vi "Read Spectrum and Save It.vi"(0 "VISA Session":refnum<visa-resource-name>, 6 "Pasta Destino DESTA aquisicao":path=path "d:/Users/Stinky/Documents", 9 "Corrente Atual (mA)":dbl, 11 "Error In":errorcluster, 12 "Iteracao":i32) -> (4 "Copy VISA Session":refnum<visa-resource-name>, 8 "PxI":dbl[](array[numeric]), 10 "XY Graph":T1(graph), 15 "Error Out":errorcluster)   [LabVIEW 2021]
uses:
  03b20bd4-ab24-4da3-90be-db98d83a5914.vi
panel:
  out "Return Data Bytes 2":u16
  out "Wavelike Data (X)":dbl[](array[numeric]) format="%.12f"
  out "Return All Data 2":string
  out "Wavelike Data (Y)":dbl[](array[numeric]) format="%.12f"
  out "Return Data Bytes":u16
  out "Return All Data":string
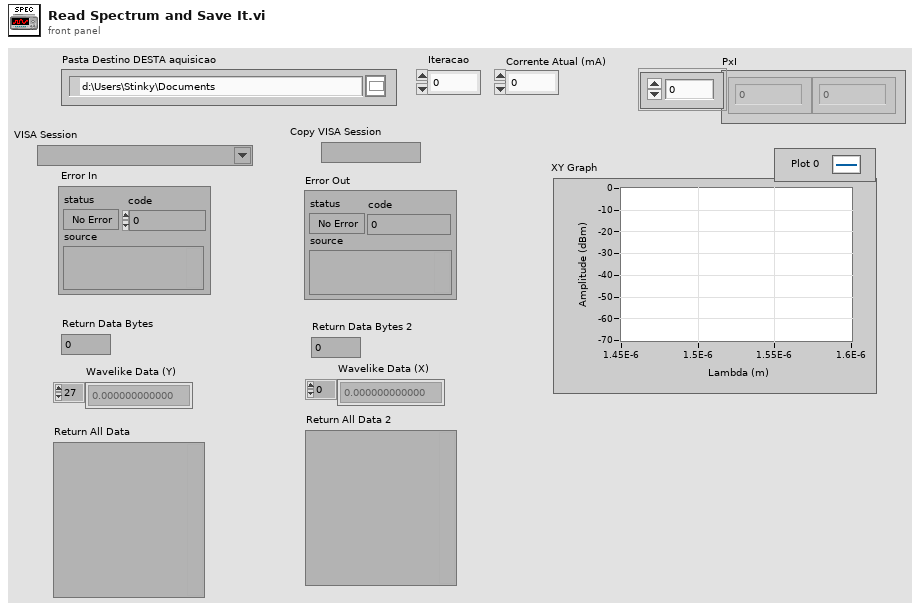
[diagram p1: front panel]
types:
  T1 = cluster{"Wavelike Data":dbl[], "Wavelike Data":dbl[]}
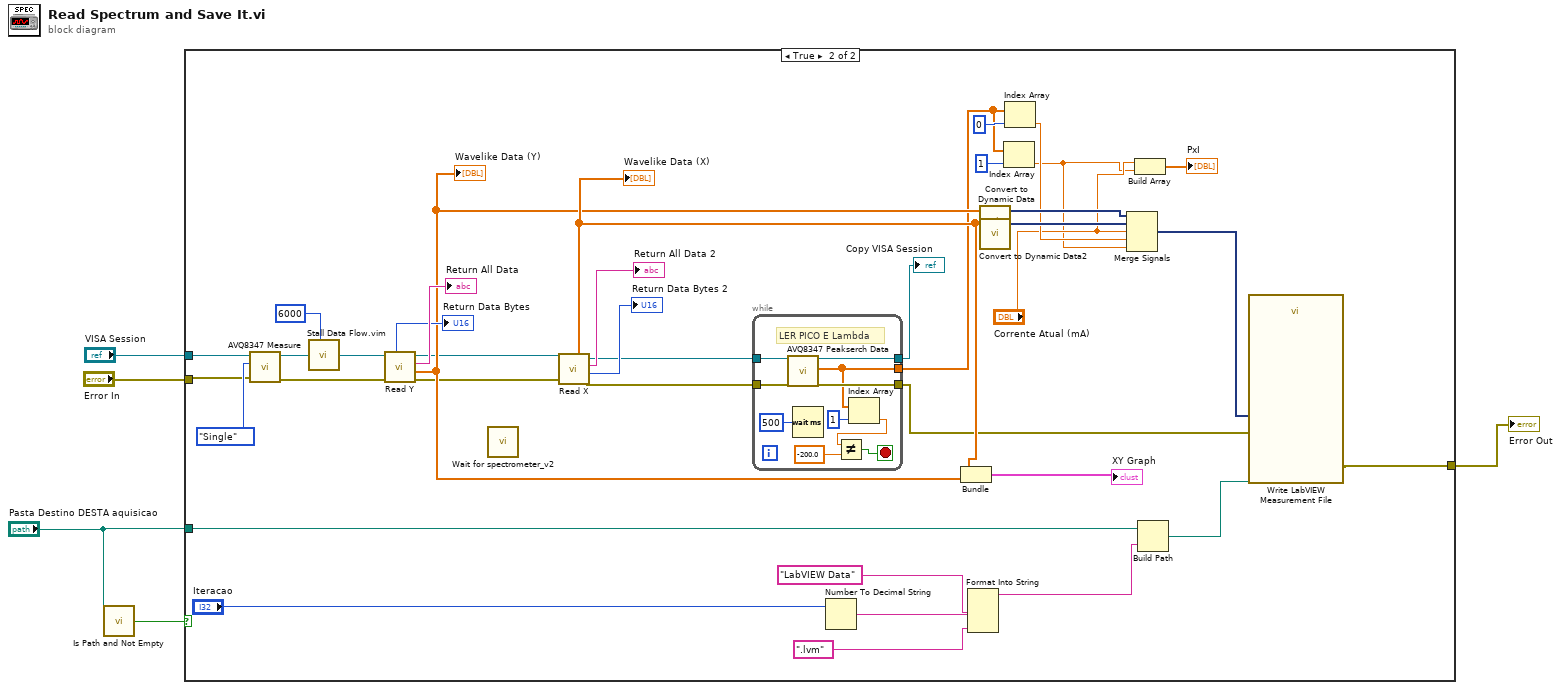
[diagram p0: block diagram]
diagram:
  n1 = call <vilib>:"Is Path and Not Empty.vi"("path"="Pasta Destino DESTA aquisicao") -> ("Is Path and Not Empty?"=w4:bool)  [unwired: 4 in]
  n2 = case shown="True" w4 {
    tunnel: "Pasta Destino DESTA aquisicao" -> [_ w37]
    tunnel: "Error In" -> [w6 w8]
    tunnel: [w6 w7] -> w2
    tunnel: "VISA Session" -> [_ w9]
    frame False {
    }
    frame True {
      n3 = call "AVQ8347 Measure.vi"("Error In"=w8, "Measure Select"=enum16{"Stop", "Single", "Repeat"}."Single", "VISA Session"=w9) -> ("Error Out"=w17:errorcluster, "Copy VISA Session"=w16:refnum<visa-resource-name>)  [unwired: 6 in, 1 out]
      n4 = call "Stall Data Flow.vim"("value in"=w16, "milliseconds to wait"=u32 6000) -> ("value out"=w15:refnum<visa-resource-name>)  [unwired: 1 out]
      n5 = call "Read Y.vi"("error in (no error)"=w17, "VISA Refnum in"=w15) -> ("error out"=w12:errorcluster, "Wavelike Data"=w35:dbl[], "Return All Data"=→"Return All Data":string, "VISA Refnum out"=w13:refnum<visa-resource-name>, "Return Data Bytes"=→"Return Data Bytes":u16)  [unwired: 5 in]
      "Wavelike Data (Y)" <- w35
      n6 = call "Wait for spectrometer_v2.vi"() -> ()  [unwired: 9 in, 3 out]
      n7 = call "Read X.vi"("error in (no error)"=w12, "VISA Refnum in"=w13) -> ("error out"=w10:errorcluster, "Return Data Bytes"=→"Return Data Bytes 2":u16, "Return All Data"=→"Return All Data 2":string, "VISA Refnum out"=w11:refnum<visa-resource-name>, "Wavelike Data"=w36:dbl[])  [unwired: 5 in]
      "Wavelike Data (X)" <- w36
      n8 = while {
        tunnel: [w48] -> w23
        tunnel: w11 -> [w52]
        tunnel: [w53] -> w27
        tunnel: w10 -> [w51]
        tunnel: [w54] -> w28
        stop <- w45 stop-if-true
        # "LER PICO E Lambda"
        n9 = call "AVQ8347 Peakserch Data.vi"("VISA Session"=w52, "Error In"=w51) -> ("Copy VISA Session"=w53:refnum<visa-resource-name>, "Peakserch Data"=w48:dbl[], "Error Out"=w54:errorcluster)  [unwired: 13 in, 2 out]
        n10 = Wait (ms)(milliseconds to wait=u32 500) -> ()  [unwired: 1 out]
        n11 = Index Array(array=w48, index=1) -> (element=w47:dbl)
        n12 = Not Equal?(x=w47, y=-200.0) -> (x != y?=w45:bool)
      }
      "Copy VISA Session" <- w27
      n13 = Number To Decimal String(number="Iteracao") -> (decimal integer string=w19:string)  [unwired: 1 in]
      n14 = Bundle("Wavelike Data"=w36, "Wavelike Data"=w35) -> (→"XY Graph":T1)  [unwired: 1 in]
      n15 = Format Into String("LabVIEW Data", w19, ".lvm") -> (resulting string=w31:string)  [unwired: 3 in, 1 out]
      n16 = call "Convert to Dynamic Data"("Array"=w35) -> ("Dynamic Data Type"=w39:dynamicdata)  [unwired: 3 in]
      n17 = call "Convert to Dynamic Data2"("Array"=w36) -> ("Dynamic Data Type"=w38:dynamicdata)  [unwired: 3 in]
      n18 = Index Array(array=w23, index=1) -> (element=w21:dbl)
      n19 = Index Array(array=w23, index=0) -> (element=w25:dbl)
      n20 = Merge Signals(w39, w38, "Corrente Atual (mA)", w25, w21) -> (w40:dynamicdata)
      n21 = Build Array("Corrente Atual (mA)", w21) -> (→"PxI":dbl[])
      n22 = Build Path(base path=w37, name or relative path=w31) -> (appended path=w29:path)
      n23 = call "Write LabVIEW Measurement File"("Signals"=w40, "error in (no error)"=w28, "Filename"=w29) -> ("error out"=w7:errorcluster)  [unwired: 14 in, 2 out]
    }
  }
  "Error Out" <- w2
